vi "TxData.vi"(7 "TxData(Hex)":string, 8 "Period(10us)":u32=100000, 9 "定时发送":bool, 10 "通道号":u8, 11 "Handle":i32) -> ()   [LabVIEW 2013]
uses:
  CHR34XXX.lvlib
panel:
  out "devId":i32
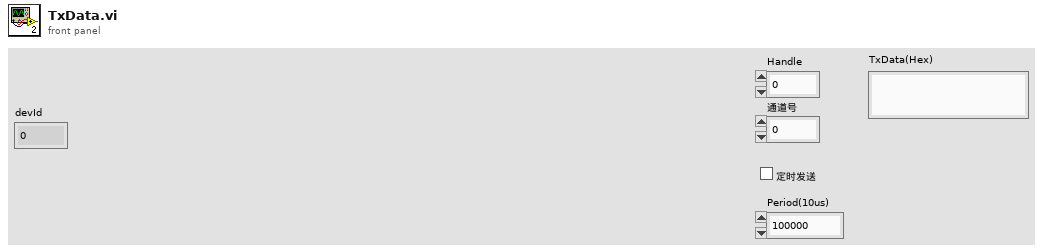
[diagram p1: front panel]
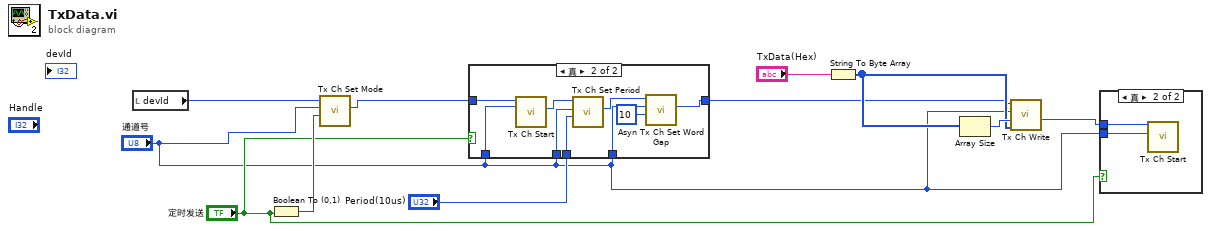
[diagram p0: block diagram]
diagram:
  n1 = local read "devId"() -> (w1:i32)
  n2 = Boolean To (0,1)(Boolean="定时发送") -> (0, 1=w10:i16)
  n3 = call "Tx Ch Set Mode.vi"("Mode"=w10, "Channel"="通道号", "devId"=w1) -> ("devId out"=w9:i32)  [unwired: 7 in, 1 out]
  n4 = case shown="真" "定时发送" {
    tunnel: w9 -> [w12 w19]
    tunnel: [w12 w13] -> w4
    tunnel: "通道号" -> [_ w21]
    tunnel: "Period(10us)" -> [_ w20]
    tunnel: "通道号" -> [_ w18]
    tunnel: "通道号" -> [_ w15]
    frame False {
    }
    frame True {
      n5 = call "Tx Ch Start.vi"("Channel"=w18, "devId"=w19) -> ("devId out"=w17:i32)  [unwired: 8 in, 1 out]
      n6 = call "Tx Ch Set Period.vi"("Period"=w20, "Channel"=w21, "devId"=w17) -> ("devId out"=w16:i32)  [unwired: 7 in, 1 out]
      n7 = call "Asyn Tx Ch Set Word Gap.vi"("Gap"=u32 10, "Channel"=w15, "devId"=w16) -> ("devId out"=w13:i32)  [unwired: 7 in, 1 out]
    }
  }
  n8 = String To Byte Array(string="TxData(Hex)") -> (unsigned byte array=w7:u8[])
  n9 = Array Size(array=w7) -> (size(s)=w8:i32)
  n10 = call "Tx Ch Write.vi"("pBuffer"=w7, "Length"=w8, "Channel"="通道号", "devId"=w4) -> ("devId out"=w3:i32)  [unwired: 5 in, 2 out]
  n11 = case shown="真" "定时发送" {
    tunnel: w3 -> [_ w23]
    tunnel: "通道号" -> [_ w22]
    frame False {
    }
    frame True {
      n12 = call "Tx Ch Start.vi"("Channel"=w22, "devId"=w23) -> ()  [unwired: 8 in, 2 out]
    }
  }
